vi "RSZVB Get Port Transfer Model State.vi"(8 "error in (no error)":errorcluster {"code" format="%.0x"}, 9 "Port (1)":i32=1, 10 "Channel (1)":i32=1, 11 "VISA session":refnum<visa-resource-name>) -> (0 "error out":errorcluster {"code" format="%.0x"}, 2 "State":bool, 3 "dup VISA session":refnum<visa-resource-name>)   [LabVIEW 2011]
doc: "This VI returns the advanced power transfer model for the converter port <Pt> state.\n\nNotes:\n(1) This command is overwritten by the general power transfer model settings; see [SENSe<Ch>:]CONVerter:AMODel.\n\nRemote-control command(s):\nSOURce<Ch>:POWer<Pt>:CONVerter:TRANsfer:AMODel?"
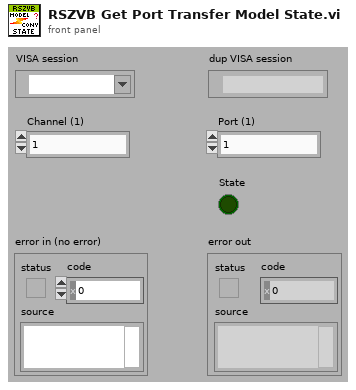
[diagram p1: front panel]
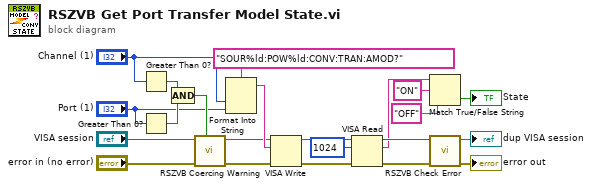
[diagram p0: block diagram]
diagram:
  n1 = Greater Than 0?(x="Channel (1)") -> (x > 0?=w18:bool)
  n2 = Greater Than 0?(x="Port (1)") -> (x > 0?=w17:bool)
  n3 = Compound Arithmetic op=AND(w18, w17) -> (w16:bool)
  n4 = call "RSZVB Coercing Warning.vi"("In Range?"=w16, "error in (no error)"="error in (no error)", "VISA session"="VISA session") -> ("error out"=w21:errorcluster, "dup VISA session"=w20:refnum<visa-resource-name>)  [unwired: 7 in]
  n5 = Format Into String(format string="SOUR%ld:POW%ld:CONV:TRAN:AMOD?", "Channel (1)", "Port (1)") -> (resulting string=w22:string)  [unwired: 2 in, 1 out]
  n6 = VISA Write(VISA resource name=w20, write buffer=w22, error in (no error)=w21) -> (VISA resource name out=w4:refnum<visa-resource-name>, error out=w5:errorcluster)  [unwired: 1 out]
  n7 = VISA Read(VISA resource name=w4, byte count=u32 1024, error in (no error)=w5) -> (VISA resource name out=w9:refnum<visa-resource-name>, read buffer=w8:string, error out=w10:errorcluster)  [unwired: 1 out]
  n8 = Match True/False String(2:"OFF" ("false string"), 3:"ON" ("true string"), 4:w8) -> (0:→"State":bool)  [unwired: 1 out]
  n9 = call "RSZVB Check Error.vi"("error in (no error)"=w10, "VISA session"=w9) -> ("error out"=→"error out":errorcluster, "dup VISA session"=→"dup VISA session":refnum<visa-resource-name>)  [unwired: 8 in]
